vi "SetParam.vi"(8 "error in (no error)":errorcluster caption="entrée d'erreur (pas d'erreur)", 10 "balanced_accuracy_score":cluster{"sample_weight":dbl[], "adjusted":bool}, 11 "Balanced_Accuracy_Score.lvclass":refnum<class "Balanced_Accuracy_Score.lvclass">) -> (0 "error out":errorcluster caption="sortie d'erreur", 3 "Balanced_Accuracy_Score.lvclass":refnum<class "Balanced_Accuracy_Score.lvclass">)   [LabVIEW 2020, in "Balanced_Accuracy_Score.lvclass"]
doc: "Set Parameters"
uses:
  Balanced_Accuracy_Score.lvclass
  Balanced_Accuracy_Score.lvclass/Balanced_Accuracy_Score.ctl
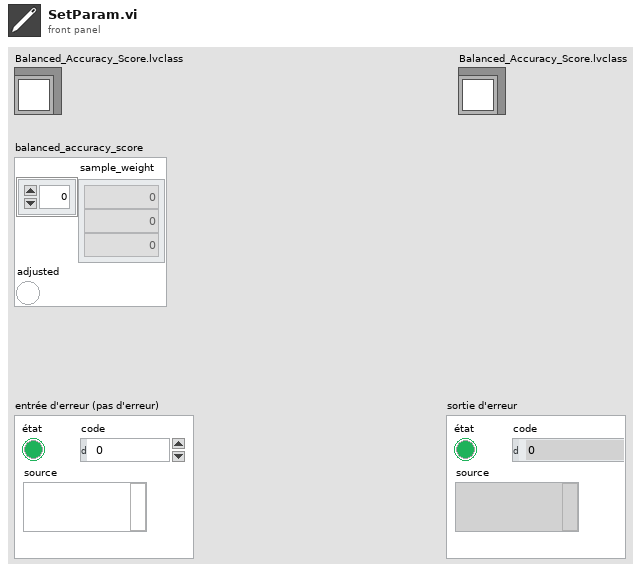
[diagram p1: front panel]
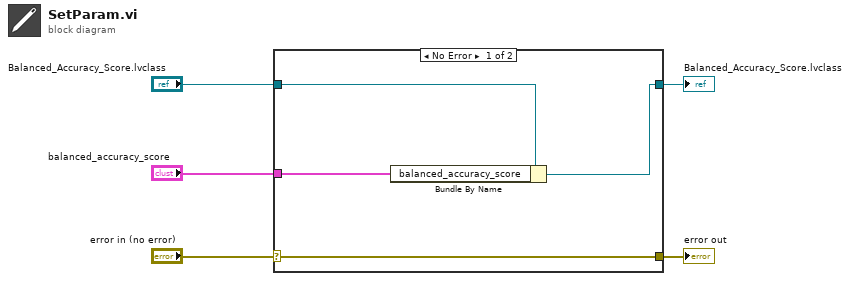
[diagram p0: block diagram]
diagram:
  n1 = case shown="No Error" "error in (no error)" {
    selector: "error in (no error)" -> [w9 w10]
    tunnel: [w9 w10] -> w4
    tunnel: [w7 w11] -> w2
    tunnel: "Balanced_Accuracy_Score.lvclass" -> [w8 w11]
    tunnel: "balanced_accuracy_score" -> [w6 _]
    frame No Error {
      n2 = Bundle By Name(cluster=w8, "balanced_accuracy_score"=w6) -> (w7:refnum<class "Balanced_Accuracy_Score.lvclass">)
    }
    frame Error {
    }
  }
  "error out" <- w4
  "Balanced_Accuracy_Score.lvclass" <- w2
